vi "Read ADC.vi"(8 "error in (no error)":errorcluster, 10 "ADC CH":dbl, 11 "Simulado in":refnum<class "Simulado.lvclass">) -> (0 "error out":errorcluster, 3 "Simulado out":refnum<class "Simulado.lvclass">)   [LabVIEW 2020, in "Simulado.lvclass"]
uses:
  Simulado.lvclass
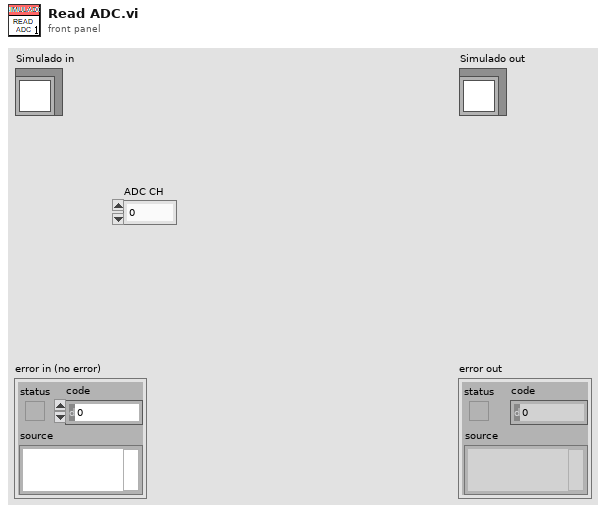
[diagram p1: front panel]
types:
  T1 = enum16{"reset parameters", "Get parameters", "Set parameter"}
  T2 = typedef "Serial Device.lvclass/serial device brand.ctl" = string
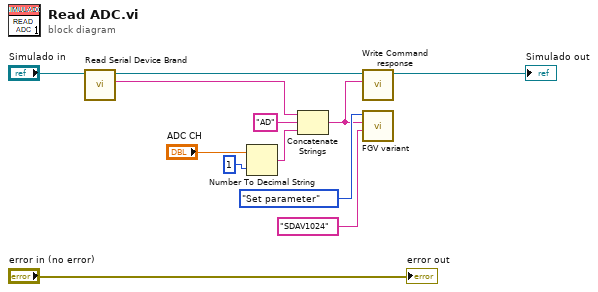
[diagram p0: block diagram]
diagram:
  n1 = call-dynamic "Read Serial Device Brand.vi"("Serial Device in"="Simulado in") -> ("Serial Device Brand"=w3:T2, "Serial Device out"=w11:refnum<class "Simulado.lvclass">)  [unwired: 8 in, 1 out]
  n2 = Number To Decimal String(number="ADC CH", width (-)=i16 1) -> (decimal integer string=w2:string)
  n3 = Concatenate Strings(w3, "AD" ("string"), w2) -> (w1:string)
  n4 = call-dynamic "Write Command response.vi"("Command response"=w1, "Simulado in"=w11) -> ("Simulado out"=→"Simulado out":refnum<class "Simulado.lvclass">)  [unwired: 8 in, 1 out]
  n5 = call "FGV variant.vi"("Response to save"="SDAV1024", "Command"=w1, "Functions"=T1."Set parameter") -> ()  [unwired: 7 in, 2 out]
  "error out" <- "error in (no error)"
